vi "Create_Trajectory_Traj_Meters_To_PW_Units.vi"(10 "States in_M":T1[](array[typedef]) {"POSE"."ROTATION"."SIN" format="%13.4f"; "POSE"."ROTATION"."COS" format="%13.4f"; "POSE"."ROTATION"."VALUE" format="%13.4f"; "POSE"."TRANSLATION"."Y" format="%14.3f"; "POSE"."TRANSLATION"."X" format="%14.3f"}, 11 "PathWeaver Length Units":T5(ring)) -> (3 "States out_UNITS":T1[](array[typedef]) {"POSE"."ROTATION"."SIN" format="%13.4f"; "POSE"."ROTATION"."COS" format="%13.4f"; "POSE"."ROTATION"."VALUE" format="%13.4f"; "POSE"."TRANSLATION"."Y" format="%14.3f"; "POSE"."TRANSLATION"."X" format="%14.3f"})   [LabVIEW 2019]
uses:
  <vilib>/Rock Robotics/WPI/ThirdParty/JAS_Junk/TrajLib/TypeDef/TRAJ_STATE.ctl
  <vilib>/Rock Robotics/WPI/ThirdParty/JAS_Junk/TrajLib/TypeDef/POSE2D.ctl
  <vilib>/Rock Robotics/WPI/ThirdParty/JAS_Junk/TrajLib/TypeDef/TRANSLATION2D.ctl
  <vilib>/Rock Robotics/WPI/ThirdParty/JAS_Junk/TrajLib/TypeDef/ROTATION2D.ctl
  <vilib>/Rock Robotics/WPI/ThirdParty/JAS_Junk/TrajLib/Trajectory_Library.lvlib
panel:
  # "Convert Meters of trajectory states  to PathWeaver UNITS"
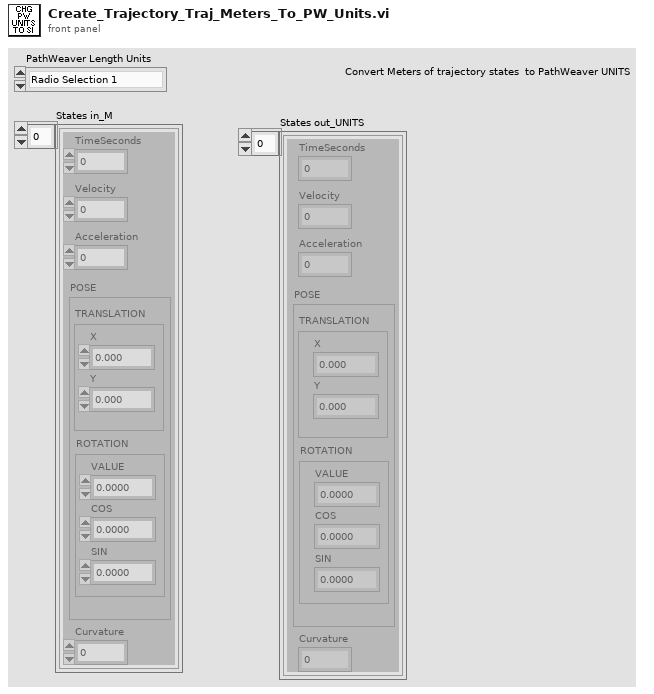
[diagram p1: front panel]
types:
  T1 = typedef "Trajectory_Library.lvlib/TRAJ_STATE.ctl" = cluster{"TimeSeconds":dbl, "Velocity":dbl, "Acceleration":dbl, "POSE":T2, "Curvature":dbl}
  T2 = typedef "Trajectory_Library.lvlib/POSE2D.ctl" = cluster{"TRANSLATION":T3, "ROTATION":T4}
  T3 = typedef "Trajectory_Library.lvlib/TRANSLATION2D.ctl" = cluster{"X":dbl, "Y":dbl}
  T4 = typedef "Trajectory_Library.lvlib/ROTATION2D.ctl" = cluster{"VALUE":dbl, "COS":dbl, "SIN":dbl}
  T5 = enum32{"Radio Selection 1", "Radio Selection 2", "Radio Selection 3", "Radio Selection 4", "Radio Selection 5"}
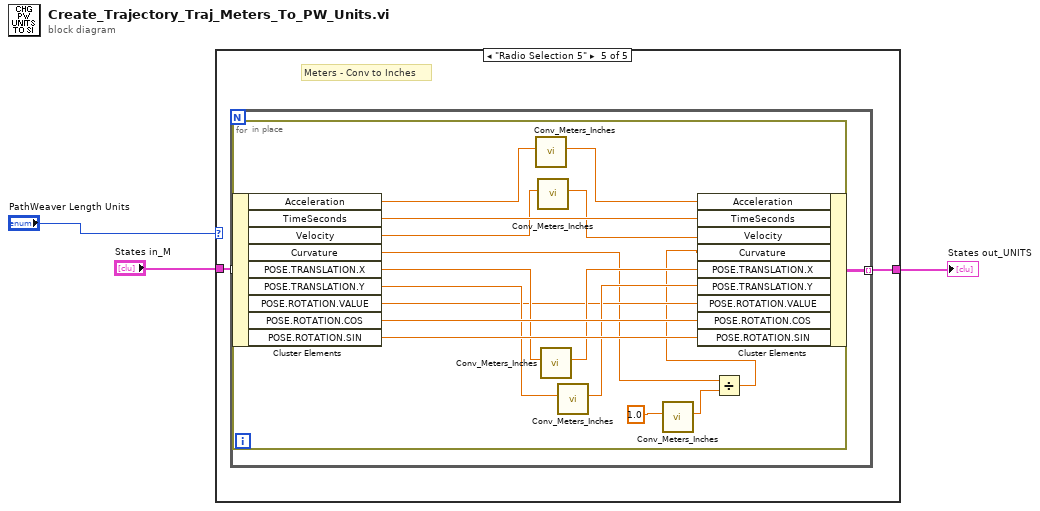
[diagram p0: block diagram]
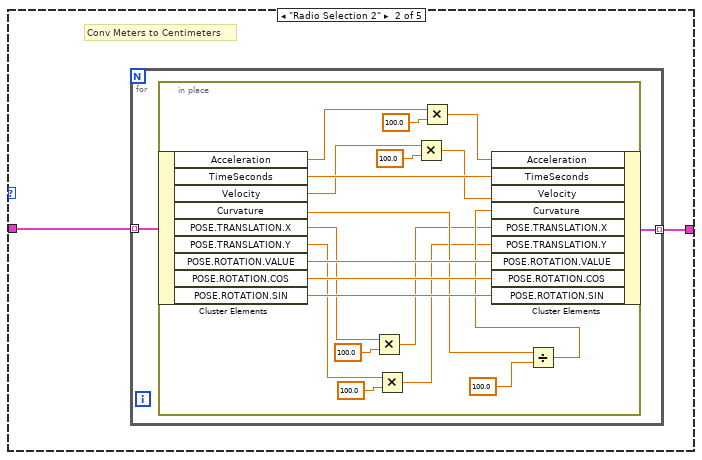
[diagram p3: hidden frame]
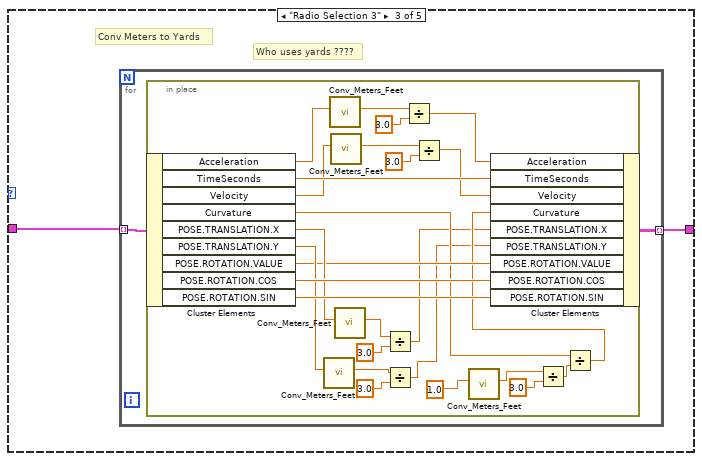
[diagram p4: hidden frame]
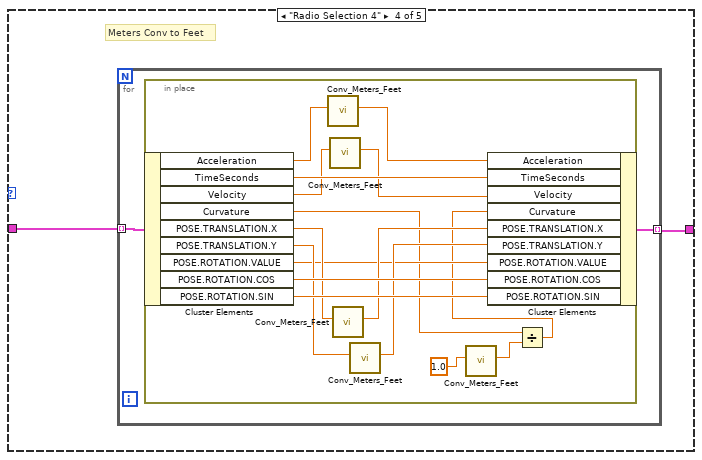
[diagram p5: hidden frame]
diagram:
  n1 = case shown="\"Radio Selection 5\"" "PathWeaver Length Units" {
    tunnel: "States in_M" -> [w4 w5 w29 w59 w79]
    tunnel: [w4 w6 w28 w58 w78] -> w3
    frame "Radio Selection 1" {
      # "Meters - do nothing"
    }
    frame "Radio Selection 2" {
      # "Conv Meters to Centimeters"
      n2 = for {
        tunnel: w5 -> [w8] mode=indexing
        tunnel: [w7] -> w6 mode=indexing
        n3 = in-place {
          n4 = in-place-cluster #1(w8) -> ("Acceleration"=w19:dbl, "TimeSeconds"=w27:dbl, "Velocity"=w17:dbl, "Curvature"=w22:dbl, "POSE.TRANSLATION.X"=w9:dbl, "POSE.TRANSLATION.Y"=w13:dbl, "POSE.ROTATION.VALUE"=w24:dbl, "POSE.ROTATION.COS"=w26:dbl, "POSE.ROTATION.SIN"=w25:dbl)
          n5 = Multiply(x=w9, y=100.0) -> (x*y=w10:dbl)
          n6 = Multiply(x=w13, y=100.0) -> (x*y=w12:dbl)
          n7 = Multiply(x=w17, y=100.0) -> (x*y=w16:dbl)
          n8 = Multiply(x=w19, y=100.0) -> (x*y=w20:dbl)
          n9 = Divide(x=w22, y=100.0 ("Centimeter")) -> (x/y=w23:dbl)
          n10 = in-place-cluster #1("Acceleration"=w20, "TimeSeconds"=w27, "Velocity"=w16, "Curvature"=w23, "POSE.TRANSLATION.X"=w10, "POSE.TRANSLATION.Y"=w12, "POSE.ROTATION.VALUE"=w24, "POSE.ROTATION.COS"=w26, "POSE.ROTATION.SIN"=w25) -> (w7:T1)
        }
      }
    }
    frame "Radio Selection 3" {
      # "Who uses yards ????"
      # "Conv Meters to Yards"
      n11 = for {
        tunnel: w29 -> [w31] mode=indexing
        tunnel: [w30] -> w28 mode=indexing
        n12 = in-place {
          n13 = in-place-cluster #2(w31) -> ("Acceleration"=w51:dbl, "TimeSeconds"=w57:dbl, "Velocity"=w52:dbl, "Curvature"=w49:dbl, "POSE.TRANSLATION.X"=w53:dbl, "POSE.TRANSLATION.Y"=w54:dbl, "POSE.ROTATION.VALUE"=w50:dbl, "POSE.ROTATION.COS"=w56:dbl, "POSE.ROTATION.SIN"=w55:dbl)
          n14 = call <vilib>:"Conv_Meters_Feet.vi"("Meters"=w54) -> ("Feet"=w36:dbl)  [unwired: 10 in]
          n15 = call <vilib>:"Conv_Meters_Feet.vi"("Meters"=w51) -> ("Feet"=w46:dbl)  [unwired: 10 in]
          n16 = call <vilib>:"Conv_Meters_Feet.vi"("Meters"=w52) -> ("Feet"=w42:dbl)  [unwired: 10 in]
          n17 = call <vilib>:"Conv_Meters_Feet.vi"("Meters"=w53) -> ("Feet"=w33:dbl)  [unwired: 10 in]
          n18 = Divide(x=w33, y=3.0) -> (x/y=w32:dbl)
          n19 = Divide(x=w36, y=3.0) -> (x/y=w35:dbl)
          n20 = Divide(x=w46, y=3.0) -> (x/y=w44:dbl)
          n21 = Divide(x=w42, y=3.0) -> (x/y=w41:dbl)
          n22 = call <vilib>:"Conv_Meters_Feet.vi"("Meters"=1.0 ("Centimeter")) -> ("Feet"=w38:dbl)  [unwired: 10 in]
          n23 = Divide(x=w38, y=3.0) -> (x/y=w39:dbl)
          n24 = Divide(x=w49, y=w39) -> (x/y=w48:dbl)
          n25 = in-place-cluster #2("Acceleration"=w44, "TimeSeconds"=w57, "Velocity"=w41, "Curvature"=w48, "POSE.TRANSLATION.X"=w32, "POSE.TRANSLATION.Y"=w35, "POSE.ROTATION.VALUE"=w50, "POSE.ROTATION.COS"=w56, "POSE.ROTATION.SIN"=w55) -> (w30:T1)
        }
      }
    }
    frame "Radio Selection 4" {
      # "Meters Conv to Feet"
      n26 = for {
        tunnel: w59 -> [w61] mode=indexing
        tunnel: [w60] -> w58 mode=indexing
        n27 = in-place {
          n28 = in-place-cluster #3(w61) -> ("Acceleration"=w69:dbl, "TimeSeconds"=w77:dbl, "Velocity"=w71:dbl, "Curvature"=w63:dbl, "POSE.TRANSLATION.X"=w73:dbl, "POSE.TRANSLATION.Y"=w74:dbl, "POSE.ROTATION.VALUE"=w66:dbl, "POSE.ROTATION.COS"=w76:dbl, "POSE.ROTATION.SIN"=w75:dbl)
          n29 = call <vilib>:"Conv_Meters_Feet.vi"("Meters"=w69) -> ("Feet"=w68:dbl)  [unwired: 10 in]
          n30 = call <vilib>:"Conv_Meters_Feet.vi"("Meters"=w71) -> ("Feet"=w70:dbl)  [unwired: 10 in]
          n31 = call <vilib>:"Conv_Meters_Feet.vi"("Meters"=w73) -> ("Feet"=w72:dbl)  [unwired: 10 in]
          n32 = call <vilib>:"Conv_Meters_Feet.vi"("Meters"=w74) -> ("Feet"=w67:dbl)  [unwired: 10 in]
          n33 = call <vilib>:"Conv_Meters_Feet.vi"("Meters"=1.0 ("Centimeter")) -> ("Feet"=w64:dbl)  [unwired: 10 in]
          n34 = Divide(x=w63, y=w64) -> (x/y=w62:dbl)
          n35 = in-place-cluster #3("Acceleration"=w68, "TimeSeconds"=w77, "Velocity"=w70, "Curvature"=w62, "POSE.TRANSLATION.X"=w72, "POSE.TRANSLATION.Y"=w67, "POSE.ROTATION.VALUE"=w66, "POSE.ROTATION.COS"=w76, "POSE.ROTATION.SIN"=w75) -> (w60:T1)
        }
      }
    }
    frame "Radio Selection 5" {
      # "Meters - Conv to Inches"
      n36 = for {
        tunnel: w79 -> [w81] mode=indexing
        tunnel: [w80] -> w78 mode=indexing
        n37 = in-place {
          n38 = in-place-cluster #4(w81) -> ("Acceleration"=w89:dbl, "TimeSeconds"=w97:dbl, "Velocity"=w91:dbl, "Curvature"=w83:dbl, "POSE.TRANSLATION.X"=w93:dbl, "POSE.TRANSLATION.Y"=w94:dbl, "POSE.ROTATION.VALUE"=w86:dbl, "POSE.ROTATION.COS"=w96:dbl, "POSE.ROTATION.SIN"=w95:dbl)
          n39 = call <vilib>:"Conv_Meters_Inches.vi"("Meters"=w89) -> ("Inches"=w88:dbl)  [unwired: 10 in]
          n40 = call <vilib>:"Conv_Meters_Inches.vi"("Meters"=w91) -> ("Inches"=w90:dbl)  [unwired: 10 in]
          n41 = call <vilib>:"Conv_Meters_Inches.vi"("Meters"=w93) -> ("Inches"=w92:dbl)  [unwired: 10 in]
          n42 = call <vilib>:"Conv_Meters_Inches.vi"("Meters"=w94) -> ("Inches"=w87:dbl)  [unwired: 10 in]
          n43 = call <vilib>:"Conv_Meters_Inches.vi"("Meters"=1.0 ("Centimeter")) -> ("Inches"=w84:dbl)  [unwired: 10 in]
          n44 = Divide(x=w83, y=w84) -> (x/y=w82:dbl)
          n45 = in-place-cluster #4("Acceleration"=w88, "TimeSeconds"=w97, "Velocity"=w90, "Curvature"=w82, "POSE.TRANSLATION.X"=w92, "POSE.TRANSLATION.Y"=w87, "POSE.ROTATION.VALUE"=w86, "POSE.ROTATION.COS"=w96, "POSE.ROTATION.SIN"=w95) -> (w80:T1)
        }
      }
    }
  }
  "States out_UNITS" <- w3
